vi "write_focus_file.vi"(5 "Log_dir":path caption="Chemin du dossier de log", 7 "Instrument":string, 8 "Foyer":dbl caption="Foyer du télescope", 9 "Temp.str":dbl caption="Temp. Serrurier" format="%.1f", 10 "Temp.int":dbl format="%.1f", 11 "Temp.ext":dbl caption="Temp. ext" format="%.1f") -> ()   [LabVIEW 2011]
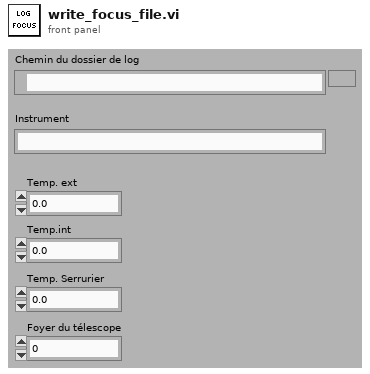
[diagram p1: front panel]
types:
  T1 = enum16{"open", "replace", "create", "open or create", "replace or create", "replace or create with confirmation"}
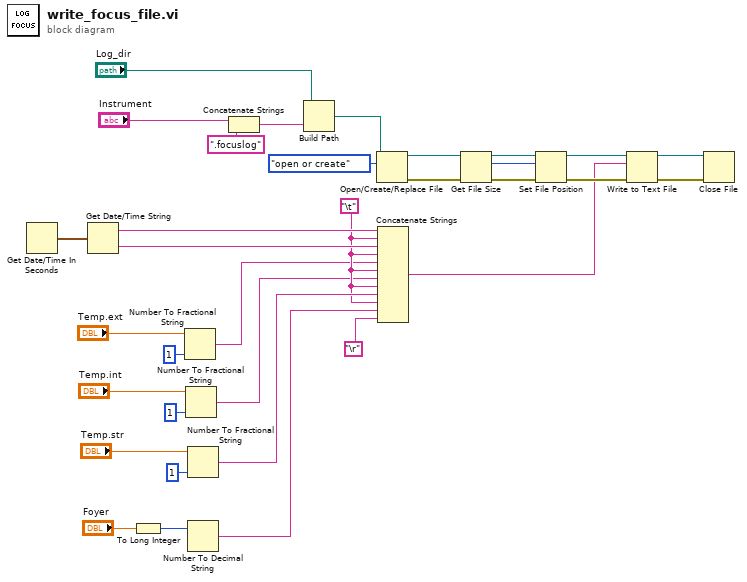
[diagram p0: block diagram]
diagram:
  w4 = "\t"
  n1 = Get Date/Time In Seconds() -> (seconds since 1Jan1904=w33:timestamp)
  n2 = Get Date/Time String(seconds (now)=w33) -> (date string=w26:string, time string=w28:string)  [unwired: 2 in]
  n3 = To Long Integer(number="Foyer") -> (32bit integer=w29:i32)
  n4 = Number To Fractional String(number="Temp.ext", precision (6)=i16 1) -> (F-format string=w2:string)  [unwired: 2 in]
  n5 = Number To Fractional String(number="Temp.int", precision (6)=i16 1) -> (F-format string=w3:string)  [unwired: 2 in]
  n6 = Number To Fractional String(number="Temp.str", precision (6)=i16 1) -> (F-format string=w5:string)  [unwired: 2 in]
  n7 = Number To Decimal String(number=w29) -> (decimal integer string=w6:string)  [unwired: 1 in]
  n8 = Concatenate Strings("Instrument", ".focuslog" ("string")) -> (w27:string)
  n9 = Build Path(base path="Log_dir", name or relative path=w27) -> (appended path=w24:path)
  n10 = Open/Create/Replace File(file path (use dialog)=w24, operation (0:open)=T1."open or create") -> (refnum out=w23:refnum<file>, error out=w22:errorcluster)  [unwired: 4 in, 1 out]
  n11 = Concatenate Strings(w26, w4, w28, w4, w2, w4, w3, w4, w5, w4, w6, "\r") -> (w17:string)
  n12 = Get File Size(file=w23, error in=w22) -> (refnum out=w21:refnum<file>, size (in bytes)=w13:i64, 0:w20:errorcluster)
  n13 = Set File Position(offset (in bytes) (0)=w13, refnum=w21, error in=w20) -> (refnum out=w19:refnum<file>, error out=w18:errorcluster)  [unwired: 1 in]
  n14 = Write to Text File(file (use dialog)=w19, text=w17, error in=w18) -> (refnum out=w16:refnum<file>, error out=w15:errorcluster)  [unwired: 1 in, 1 out]
  n15 = Close File(refnum=w16, error in=w15) -> ()  [unwired: 2 out]
